vi "Write User Interface.lvclass.vi"(8 "error in (no error)":errorcluster, 10 "User Interface.lvclass":refnum<class "UI.lvclass">, 11 "Launch UI Message in":refnum<class "Launch User Interface Msg.lvclass">) -> (0 "error out":errorcluster, 3 "Launch UI Message out":refnum<class "Launch User Interface Msg.lvclass">)   [LabVIEW 2026, in "Controller Actor.lvlib" / "Launch User Interface Msg.lvclass"]
uses:
  Launch User Interface Msg.lvclass
  Launch User Interface Msg.lvclass/Launch User Interface Msg.ctl
  User Interface/UI.lvclass
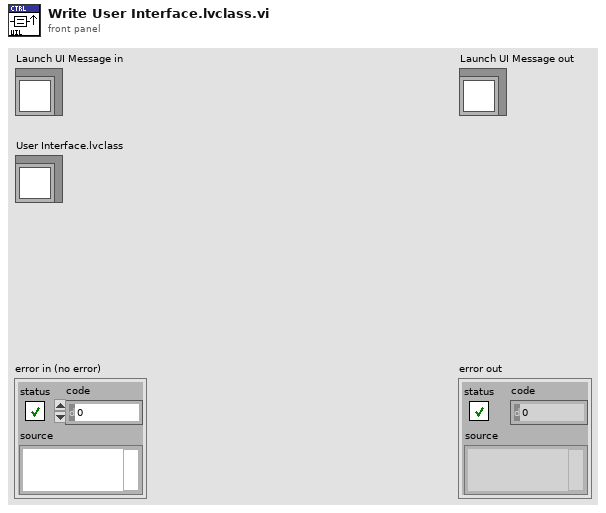
[diagram p1: front panel]
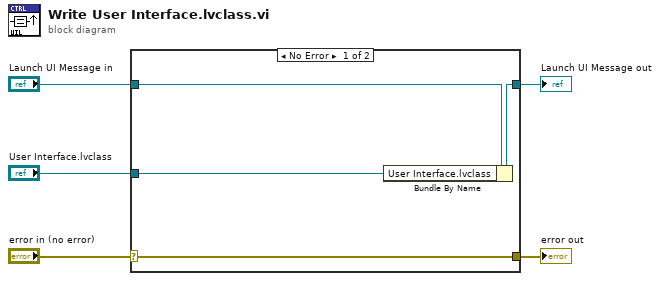
[diagram p0: block diagram]
diagram:
  n1 = case shown="No Error" "error in (no error)" {
    selector: "error in (no error)" -> [w9 w10]
    tunnel: [w9 w10] -> w4
    tunnel: [w7 w11] -> w2
    tunnel: "Launch UI Message in" -> [w8 w11]
    tunnel: "User Interface.lvclass" -> [w6 _]
    frame No Error {
      n2 = Bundle By Name(cluster=w8, "User Interface.lvclass"=w6) -> (w7:refnum<class "Launch User Interface Msg.lvclass">)
    }
    frame Error {
    }
  }
  "error out" <- w4
  "Launch UI Message out" <- w2
